vi "Ox_TempOnly_ITC503_LKS370.vi"() -> ()   [LabVIEW 2014]
uses:
  <vilib>/Utility/file.llb/Write To Spreadsheet File (DBL).vi
  Lake Shore Cryotronics 370/Lake Shore Cryotronics 370.lvlib
panel:
  in  "Abort!":bool
  out "Timestamp":dbl format="%#_13g"
  in  "Tab Control":enum32{"Set Up", "DATA"}(tab)
  in  "LKS370":refnum<visa-resource-name>
  in  "SampleName":string
  in  "OxfordITC503s":refnum<visa-resource-name>
  in  "error in (no error)":errorcluster
  out "XY Graph 4":cluster{dbl, dbl}[](graph) caption="SRS1"
  out "XY Graph 5":cluster{dbl, dbl}[](graph) caption="SRS1"
  out "XY Graph 6":cluster{dbl, dbl}[](graph) caption="SRS1"
  out "XY Graph 7":cluster{dbl, dbl}[](graph) caption="SRS1"
  out "Data is being stored here":string
  # "RealTime Data"
  # "Thermometry"
  # "INSTRUMENT ADDRESSES"
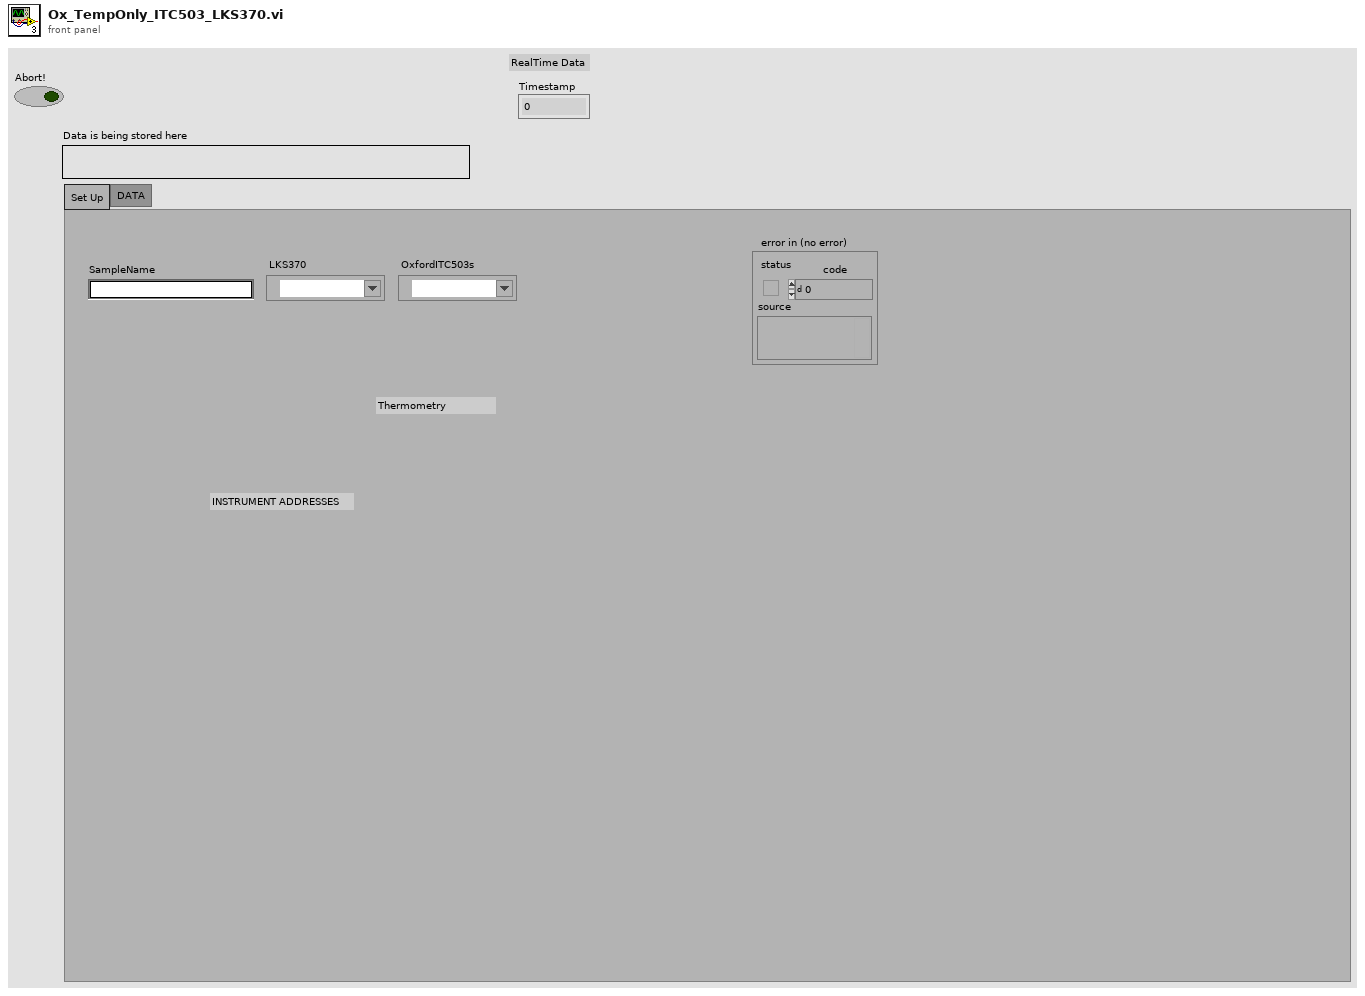
[diagram p1: front panel]
types:
  T1 = cluster{"Elapsed Time (s)":dbl, "Output of Read":dbl}
  T2 = cluster{"Elapsed Time (s)":dbl, "Resistance Reading":dbl}
  T3 = cluster{"Elapsed Time (s)":dbl, "Kelvin Reading":dbl}
  T4 = cluster{"Elapsed Time (s)":dbl, "Output of Read":dbl}[]
  T5 = cluster{"Elapsed Time (s)":dbl, "Resistance Reading":dbl}[]
  T6 = cluster{"Elapsed Time (s)":dbl, "Kelvin Reading":dbl}[]
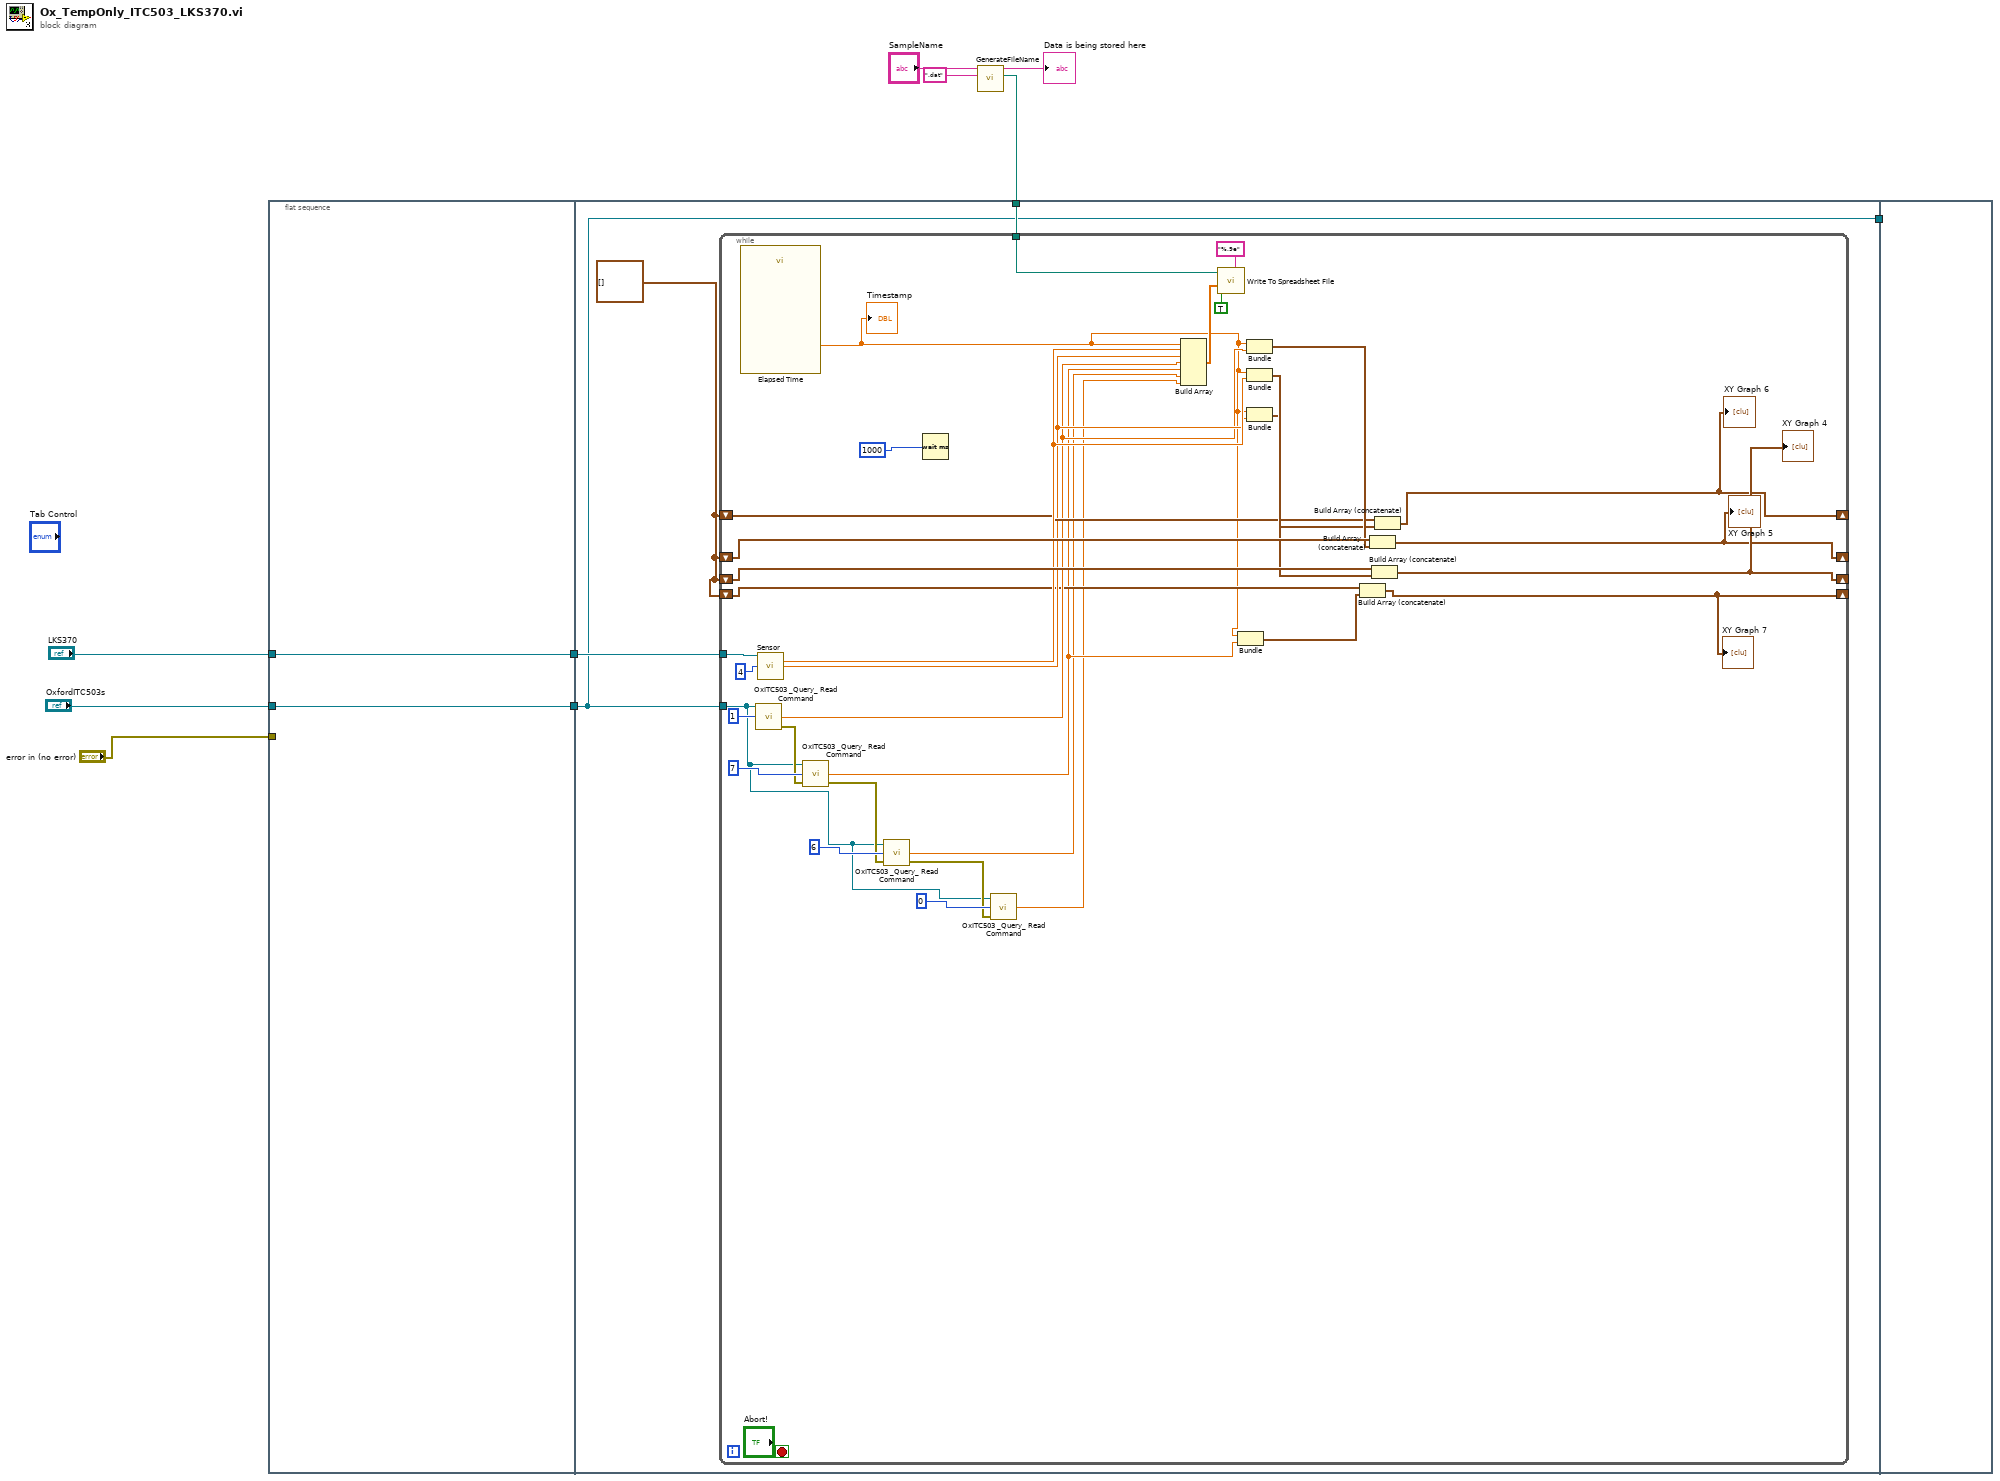
[diagram p0: block diagram]
diagram:
  n1 = flat-sequence {
    tunnel: "LKS370" -> [w12]
    tunnel: [w12] -> w6
    tunnel: [w11] -> w4
    tunnel: "OxfordITC503s" -> [w11]
    tunnel: "error in (no error)" -> [_]
    tunnel: w6 -> [w16]
    tunnel: w5 -> [w15]
    tunnel: w4 -> [w14]
    tunnel: [w14] -> w2
    tunnel: w2 -> [_]
    frame #0 {
    }
    frame #1 {
      w13 = cluster{"T1":dbl, "Elapsed Time (s)":dbl}[] []
      n2 = while {
        tunnel: w16 -> [w46]
        tunnel: w15 -> [w47]
        shift-right: [w42] -> _
        shift-left: w13 -> [w44]
        tunnel: w14 -> [w18]
        shift-right: [w41] -> _
        shift-left: w13 -> [w45]
        shift-right: [w32] -> _
        shift-left: w13 -> [w35]
        shift-right: [w28] -> _
        shift-left: w13 -> [w27]
        stop <- "Abort!" stop-if-true
        n3 = call "Elapsed Time"() -> ("Elapsed Time (s)"=w25:dbl)  [unwired: 12 in, 7 out]
        "Timestamp" <- w25
        n4 = call "OxITC503 _Query_ Read Command.vi"("Read Item"=1, "VISA session"=w18) -> ("error out (no error)"=w29:errorcluster, "Output of Read"=w31:dbl)  [unwired: 1 in, 1 out]
        n5 = call "Sensor.vi"("VISA resource name"=w46, "Channel (1)"=4) -> ("Resistance Reading"=w39:dbl, "Kelvin Reading"=w33:dbl)  [unwired: 9 in, 3 out]
        n6 = call "OxITC503 _Query_ Read Command.vi"("error in"=w29, "Read Item"=7, "VISA session"=w18) -> ("error out (no error)"=w22:errorcluster, "Output of Read"=w24:dbl)  [unwired: 1 out]
        n7 = call "OxITC503 _Query_ Read Command.vi"("error in"=w22, "Read Item"=6, "VISA session"=w18) -> ("error out (no error)"=w19:errorcluster, "Output of Read"=w21:dbl)  [unwired: 1 out]
        n8 = Wait (ms)(milliseconds to wait=1000) -> ()  [unwired: 1 out]
        n9 = call "OxITC503 _Query_ Read Command.vi"("error in"=w19, "Read Item"=0, "VISA session"=w18) -> ("Output of Read"=w17:dbl)  [unwired: 2 out]
        n10 = Build Array(w25, w39, w33, w31, w24, w21, w17) -> (w50:dbl[])
        n11 = call-poly <vilib>:"Write To Spreadsheet File.vi"("format (%.3f)"="%.9e", "append to file? (new file:F)"=TRUE, "1D data"=w50, "file path (dialog if empty)"=w47) -> ()  [unwired: 4 in, 1 out]
        n12 = Bundle("Elapsed Time (s)"=w25, "Output of Read"=w24) -> (w26:T1)  [unwired: 1 in]
        n13 = Bundle("Elapsed Time (s)"=w25, "Output of Read"=w31) -> (w38:T1)  [unwired: 1 in]
        n14 = Bundle("Elapsed Time (s)"=w25, "Resistance Reading"=w39) -> (w43:T2)  [unwired: 1 in]
        n15 = Bundle("Elapsed Time (s)"=w25, "Kelvin Reading"=w33) -> (w34:T3)  [unwired: 1 in]
        n16 = Build Array (concatenate)(w27, w26) -> (w28:T4)
        "XY Graph 7" <- w28
        n17 = Build Array (concatenate)(w45, w38) -> (w41:T4)
        "XY Graph 5" <- w41
        n18 = Build Array (concatenate)(w44, w43) -> (w42:T5)
        "XY Graph 4" <- w42
        n19 = Build Array (concatenate)(w35, w34) -> (w32:T6)
        "XY Graph 6" <- w32
      }
    }
    frame #2 {
    }
  }
  n20 = call "GenerateFileName.vi"("FileExtension"=".dat", "SampleName"="SampleName") -> ("FilePathOut"=w5:path, "FolderNameString"=→"Data is being stored here":string)  [unwired: 3 in, 1 out]
